vi "softwareTriggerInstructionHP.vi"(8 "error in (no error)":errorcluster, 10 "ModbusBuffer in":refnum<class "ModbusBuffer.lvclass">, 11 "ILCCommunications in":refnum<class "ILCCommunications.lvclass">) -> (0 "error out":errorcluster, 2 "ModbusBuffer out":refnum<class "ModbusBuffer.lvclass">, 3 "ILCCommunications out":refnum<class "ILCCommunications.lvclass">)   [LabVIEW 2016, in "ILCCommunications.lvclass"]
uses:
  ILCCommunications.lvclass
  Common_RT_Modbus/ModbusBuffer/ModbusBuffer.lvclass
  Common_RT_Modbus/ModbusBuffer/ModbusBuffer.lvclass/ModbusBuffer.ctl
  Common_RT_Modbus/ModbusBuffer/writeSoftwareTrigger.vi
  Common_RT_Modbus/ModbusBuffer/writeHeader.vi
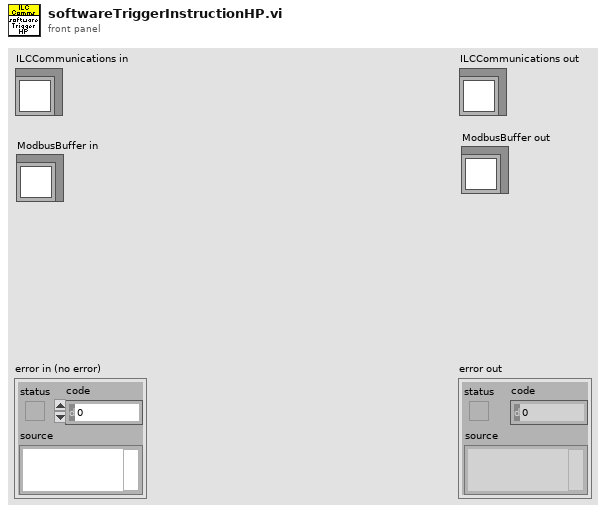
[diagram p1: front panel]
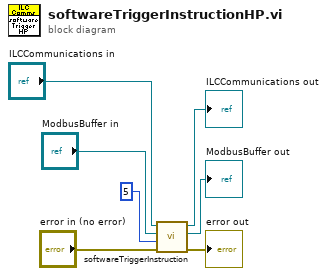
[diagram p0: block diagram]
diagram:
  n1 = call "softwareTriggerInstruction.vi"("error in (no error)"="error in (no error)", "Subnet"=u8 5, "ModbusBuffer in"="ModbusBuffer in", "ILCCommunications in"="ILCCommunications in") -> ("error out"=→"error out":errorcluster, "ModbusBuffer out"=→"ModbusBuffer out":refnum<class "ModbusBuffer.lvclass">, "ILCCommunications out"=→"ILCCommunications out":refnum<class "ILCCommunications.lvclass">)  [unwired: 5 in]
